vi "Compare Calls.vi"(8 "error in (no error)":errorcluster, 9 "VI Call 2":refnum<class "VI Call.lvclass">, 10 "VI Call 1":refnum<class "VI Call.lvclass">, 11 "String Argument Matching Comparator in":refnum<class "Matching String Input Comparator.lvclass">) -> (0 "error out":errorcluster, 1 "Description":string, 2 "Equal?":bool)   [LabVIEW 2020, in "Matching String Input Comparator.lvclass"]
uses:
  Matching String Input Comparator.lvclass
  Core/VI Call/VI Call.lvclass
  Core/Comparator/Describe Variant.vi
  astemes-string-diff-utils/source/Diff Tool.vi
  <vilib>/Utility/Data Type/NI_Data Type.lvlib
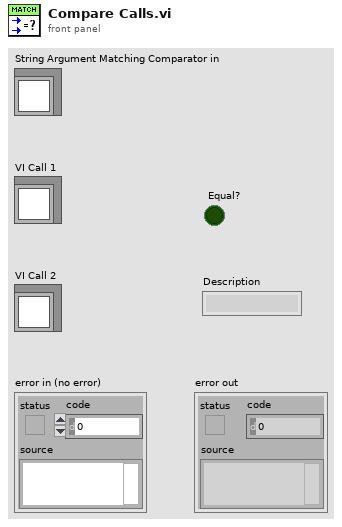
[diagram p1: front panel]
types:
  T1 = typedef "NI_Data Type.lvlib/Data Type.ctl" = enum8{"Invalid Type", "Void", "I8", "I16", "I32", "I64", "U8", "U16", "U32", "U64", "Single Float", "Double Float", "Extended Float", "Single Complex", "Double Complex", "Extended Complex", "Enum U8", "Enum U16", "Enum U32", "Enum U64", "Single Float With Unit", "Double Float With Unit", "Extended Float With Unit", "Single Complex with Unit", "Double Complex with Unit", "Extended Complex with Unit", "Boolean", "String", "Path", "Picture", "Tag", "Array", "Cluster", "Variant", "LV Variant", "Waveform", "Timestamp", "Digital Waveform", "Digital Data", "ExpressData", "Refnum", "External Data", "VI", "Poly VI", "LabVIEW Class Instance", "Fixed Point", "Set Collection", "Map Collection"}
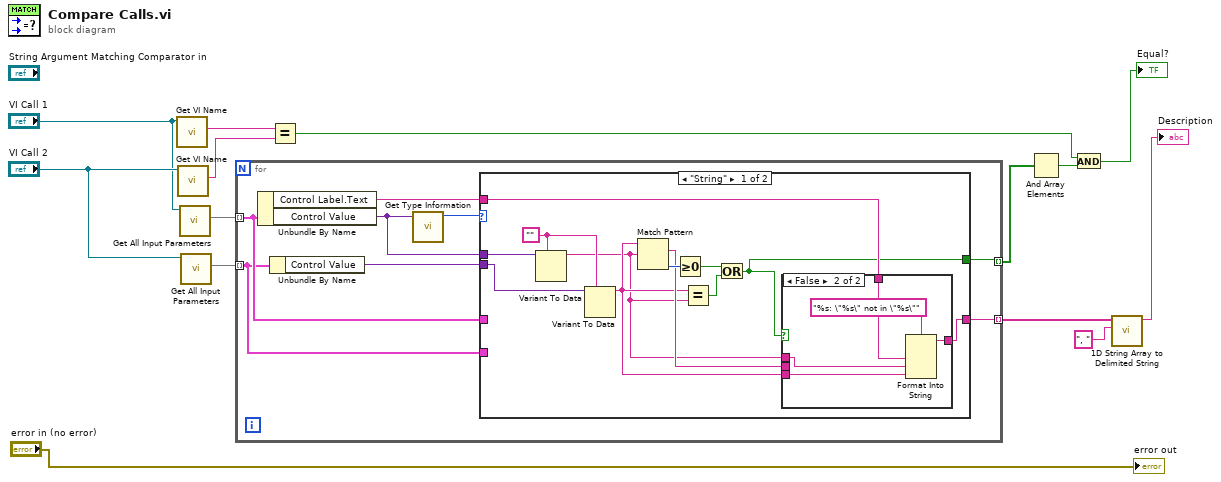
[diagram p0: block diagram]
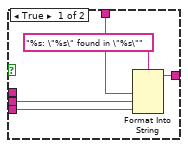
[diagram p2: hidden frame]
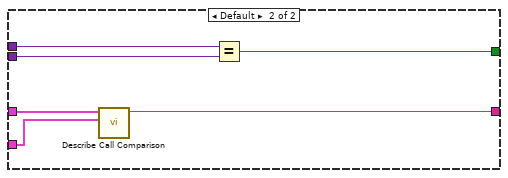
[diagram p3: hidden frame]
diagram:
  n1 = call-dynamic "Get VI Name.vi"("VI Call In"="VI Call 1") -> ("VI Name"=w9:string)  [unwired: 10 in]
  n2 = call-dynamic "Get VI Name.vi"("VI Call In"="VI Call 2") -> ("VI Name"=w8:string)  [unwired: 10 in]
  n3 = call-dynamic "Get All Input Parameters.vi"("VI Call in"="VI Call 1") -> ("Input Parameters"=w14:map{string, variant})  [unwired: 9 in, 1 out]
  n4 = call-dynamic "Get All Input Parameters.vi"("VI Call in"="VI Call 2") -> ("Input Parameters"=w13:map{string, variant})  [unwired: 9 in, 1 out]
  n5 = for {
    tunnel: w14 -> [w16] mode=indexing
    tunnel: w13 -> [w15] mode=indexing
    tunnel: [w22] -> w11 mode=indexing
    tunnel: [w18] -> w2 mode=indexing
    n6 = Unbundle By Name(w16) -> ("Control Label.Text"=w17:string, "Control Value"=w20:variant)
    n7 = Unbundle By Name(w15) -> ("Control Value"=w21:variant)
    n8 = call <vilib>:"Get Type Information.vi"("variant"=w20) -> ("type"=w19:T1)  [unwired: 6 in, 4 out]
    n9 = case shown="\"String\"" w19 {
      tunnel: [w26 w50] -> w22
      tunnel: w21 -> [w33 w49]
      tunnel: w20 -> [w34 w48]
      tunnel: w15 -> [_ w45]
      tunnel: w16 -> [_ w47]
      tunnel: [w29 w46] -> w18
      tunnel: w17 -> [w30 _]
      frame "String" {
        w32 = ""
        n10 = Variant To Data(type=w32, Variant=w34) -> (data=w24:string)  [unwired: 1 in, 1 out]
        n11 = Variant To Data(type=w32, Variant=w33) -> (data=w25:string)  [unwired: 1 in, 1 out]
        n12 = Match Pattern(string=w25, regular expression=w24) -> (match substring=w28:string, offset past match=w31:i32)  [unwired: 1 in, 2 out]
        n13 = Greater Or Equal To 0?(x=w31) -> (x >= 0?=w27:bool)
        n14 = Equal?(x=w25, y=w24) -> (x = y?=w23:bool)
        n15 = Or(x=w27, y=w23) -> (x .or. y?=w26:bool)
        n16 = case shown="False" w26 {
          tunnel: w30 -> [w38 w43]
          tunnel: [w37 w42] -> w29
          tunnel: w25 -> [w36 w41]
          tunnel: w28 -> [w35 _]
          tunnel: w24 -> [_ w40]
          frame True {
            n17 = Format Into String(format string="%s: \"%s\" found in \"%s\"", w38, w35, w36) -> (resulting string=w37:string)  [unwired: 2 in, 1 out]
          }
          frame False {
            n18 = Format Into String(format string="%s: \"%s\" not in \"%s\"", w43, w40, w41) -> (resulting string=w42:string)  [unwired: 2 in, 1 out]
          }
        }
      }
      frame Default {
        n19 = call "Describe Call Comparison.vi"("VI Call 2"=w45, "VI Call 1"=w47) -> ("delimited string"=w46:string)  [unwired: 9 in]
        n20 = Equal?(x=w48, y=w49) -> (x = y?=w50:bool)
      }
    }
  }
  n21 = Equal?(x=w9, y=w8) -> (x = y?=w6:bool)
  n22 = And Array Elements(Boolean array=w11) -> (logical AND=w10:bool)
  n23 = And(x=w6, y=w10) -> (x .and. y?=→"Equal?":bool)
  n24 = call <vilib>:"1D String Array to Delimited String.vi"("delimiter"=", ", "string array"=w2) -> ("delimited string"=→"Description":string)  [unwired: 9 in]
  "error out" <- "error in (no error)"
